vi "utility-flip-stage.vi"(1 "axis in":dbl, 2 "flip":bool) -> (0 "axis out":dbl)   [LabVIEW 2017]
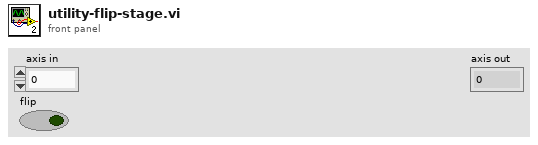
[diagram p1: front panel]
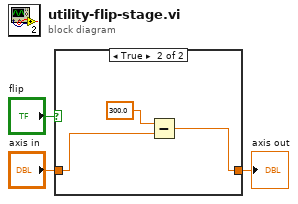
[diagram p0: block diagram]
diagram:
  n1 = case shown="True" "flip" {
    tunnel: "axis in" -> [w4 w6]
    tunnel: [w4 w5] -> w2
    frame False {
    }
    frame True {
      n2 = Subtract(x=300.0, y=w6) -> (x-y=w5:dbl)
    }
  }
  "axis out" <- w2
